vi "RunTest.vi"(8 "error in (no error)":errorcluster, 11 "Prueba09 in":refnum<class "Prueba09.lvclass">) -> (0 "error out":errorcluster, 2 "resultado":string, 3 "Prueba09 out":refnum<class "Prueba09.lvclass">)   [LabVIEW 2019, in "Prueba09.lvclass"]
uses:
  Prueba09.lvclass
  Prueba04/Control/Slide.ctl
  Prueba09.lvclass/Prueba09.ctl
  ClusterGEN.ctl
  <vilib>/Utility/miscctls.llb/LVRowAndColumnTypeDef.ctl
  <vilib>/Utility/error.llb/DialogType.ctl
  QMH/Message Queue/Enqueue Message (Single).vi
  <vilib>/Utility/error.llb/Error Cluster From Error Code.vi
  <vilib>/ErrorRing/Error Ring.xnode
  Prueba/Prueba.lvclass
  QMH/User Event - Stop/User Event - Stop.lvlib
  QMH/Message Queue/Message Queue.lvlib
  Prueba04/Prueba04.lvclass
panel:
  out "elapsed time":dbl
  out "cuenta":i32
  out "tablaPeakRef[dB]":string[](array[string])
  out "Vref2":dbl
  out "Pict Ring 2":u16(ring)
  out "Pict Ring 3":u16(ring)
  out "cumple_no_cumple":bool
  out "Vref":dbl
  in  "Tab":enum32{"Page 1", "Page 2", "Page 3"}(tab)
  out "NivMaxCpeak":dbl
  out "NivelRMSensayo":dbl
  out "frecuencia1":dbl
  in  "guardar_Vref":bool
  in  "generar1":bool
  in  "AjusteAmp":T1=40.0 caption="Ajuste de amplitud [mV]" scale=0.0..6000.0
  out "voltMon1":dbl format="%#.1f"
  out "frecMon1":dbl format="%#.1f"
  in  "seguir":bool
  out "NivMaxCpeak2":dbl
  out "NivelRMSensayo2":dbl
  out "frecuencia2":dbl
  in  "guardar_Vref2":bool
  in  "generar2":bool
  in  "AjusteAmp2":T1=40.0 caption="Ajuste de amplitud [mV]" scale=0.0..6000.0
  out "voltMon2":dbl format="%#.1f"
  out "frecMon2":dbl format="%#.1f"
  in  "seguir2":bool
  out "Pict Ring 4":u16(ring)
  out "Pict Ring 1":u16(ring)
  out "led":bool
  in  "knobFrec":dbl(knob)=1.0 min=1.0 max=3.0 scale=1.0..3.0
  in  "genera3":bool caption="PruebaSup"
  out "voltMon500":dbl format="%.1f"
  out "nivelRMS500":dbl format="%#.1f"
  in  "Tabla":string[][](table)
  in  "salir":bool
  out "cumple":bool
  out "no_cumple":bool
  out "voltMon8000":dbl format="%#.1f"
  out "nivelRM8000":dbl format="%#.1f"
  # "5550"
  # "3950"
  # "Selección de Señal de referencia 8000 Hz"
  # "Elección Señal de Referencia\nsegún marca y modelo de sonómetro"
  # "Nivel RMS para Ensayo"
  # "Nivel Máximo Cpeak"
  # "Frecuencia"
  # "Monitoreo"
  # "Frecuencia"
  # "Hz"
  # "Voltaje"
  # "mV"
  # "9. Nivel de sonido con ponderación Cpeak. IEC 61672-3: 2006 Cláusula 17"
  # "Selección de Señal de referencia 500 Hz"
  # "Elección Señal de Referencia\nsegún marca y modelo de sonómetro"
  # "Nivel RMS para Ensayo"
  # "Nivel Máximo Cpeak"
  # "Frecuencia"
  # "Monitoreo"
  # "Frecuencia"
  # "Hz"
  # "Voltaje"
  # "mV"
  # "9. Nivel de sonido con ponderación Cpeak. IEC 61672-3: 2006 Cláusula 17"
  # "Tabla Resultados"
  # "Genera peak"
  # "Cumple"
  # "No Cumple"
  # "500 Hz"
  # "Nivel RMS para Ensayo"
  # "dB"
  # "Voltaje"
  # "mV"
  # "9. Nivel de sonido con ponderación Cpeak. IEC 61672-3: 2006 Cláusula 17"
  # "8000 Hz"
  # "Nivel RMS para Ensayo"
  # "dB"
  # "Voltaje"
  # "mV"
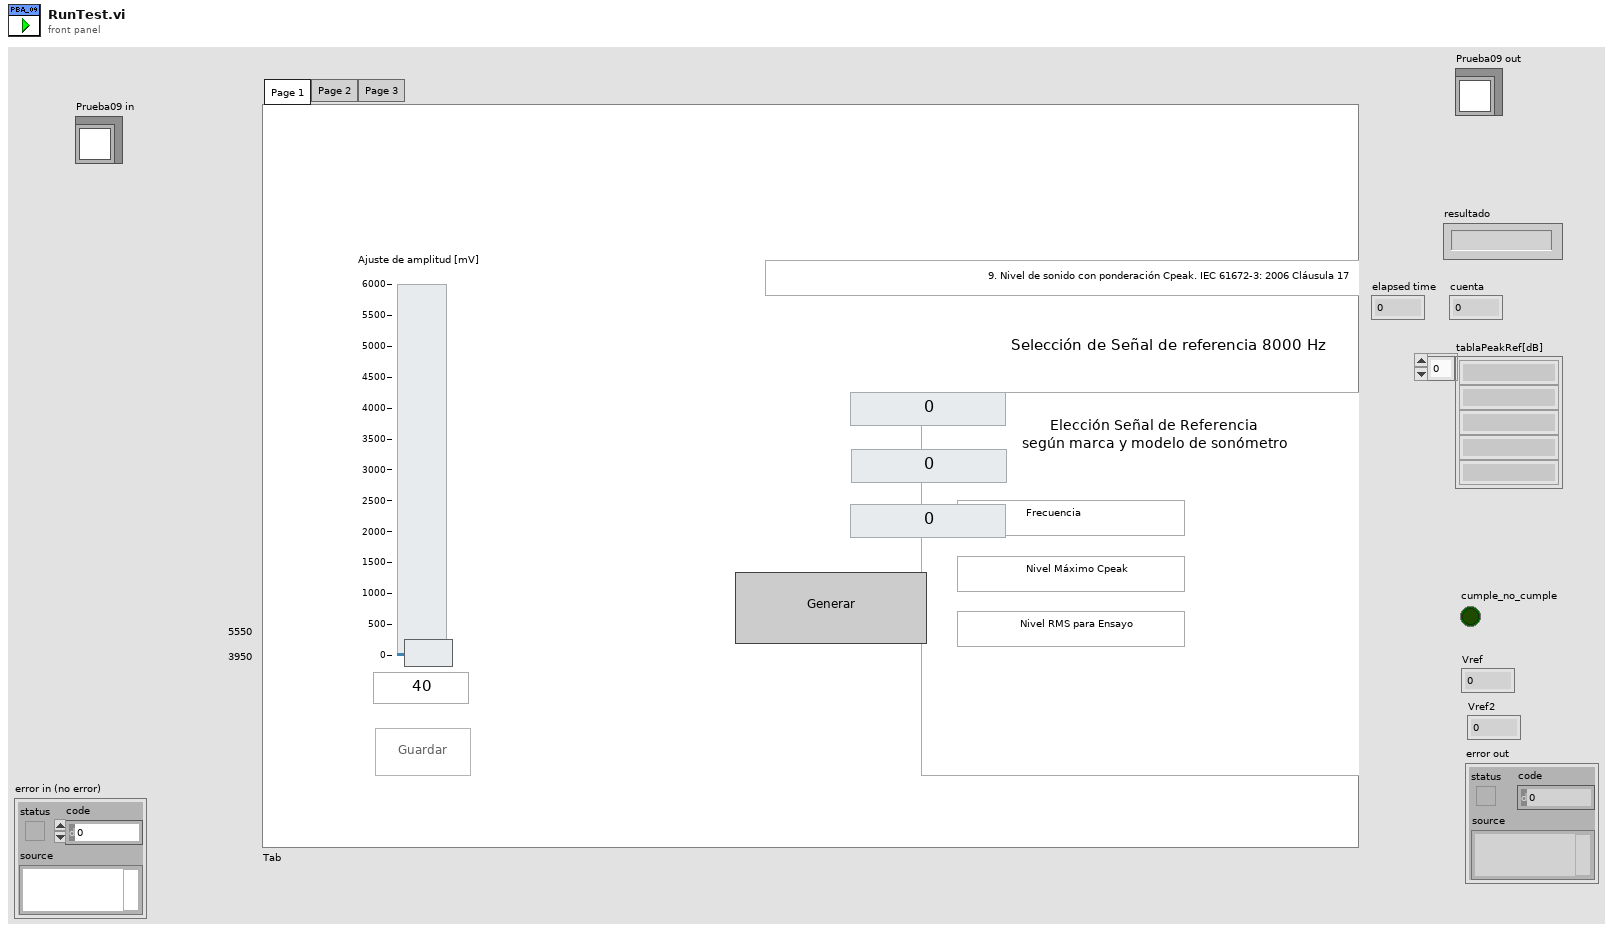
[diagram p1: front panel]
types:
  T1 = typedef "Prueba04.lvclass/Slide.ctl" = dbl
  T2 = typedef "LVRowAndColumnTypeDef.ctl" = cluster{"Row":i32, "Column":i32}
  T3 = typedef "Message Queue.lvlib/All Message Queues.ctl" = cluster{"MHL":refnum<queue>, "Inst_CNT90":refnum<queue>, "Inst_DS360":refnum<queue>, "Inst_Keithley2002":refnum<queue>, "Inst_DAQ":refnum<queue>, "BD":refnum<queue>, "Pistofono":refnum<queue>, "Nexus":refnum<queue>}
  T4 = enum8{"Enabled", "Disabled", "Disabled and Grayed Out"}
  T5 = enum32{"Page 1", "Page 2", "Page 3", "Page 4", "Page 5", "Page 6", "Page 7"}
  T6 = typedef "Prueba09.lvclass/ClusterGEN.ctl" = cluster{"frec":dbl, "amp":dbl, "tipo_ciclo":string}
  T7 = cluster{"ControlName":string, "ControlReference":refnum<vi>}[]
  T8 = typedef "DialogType.ctl" = u16
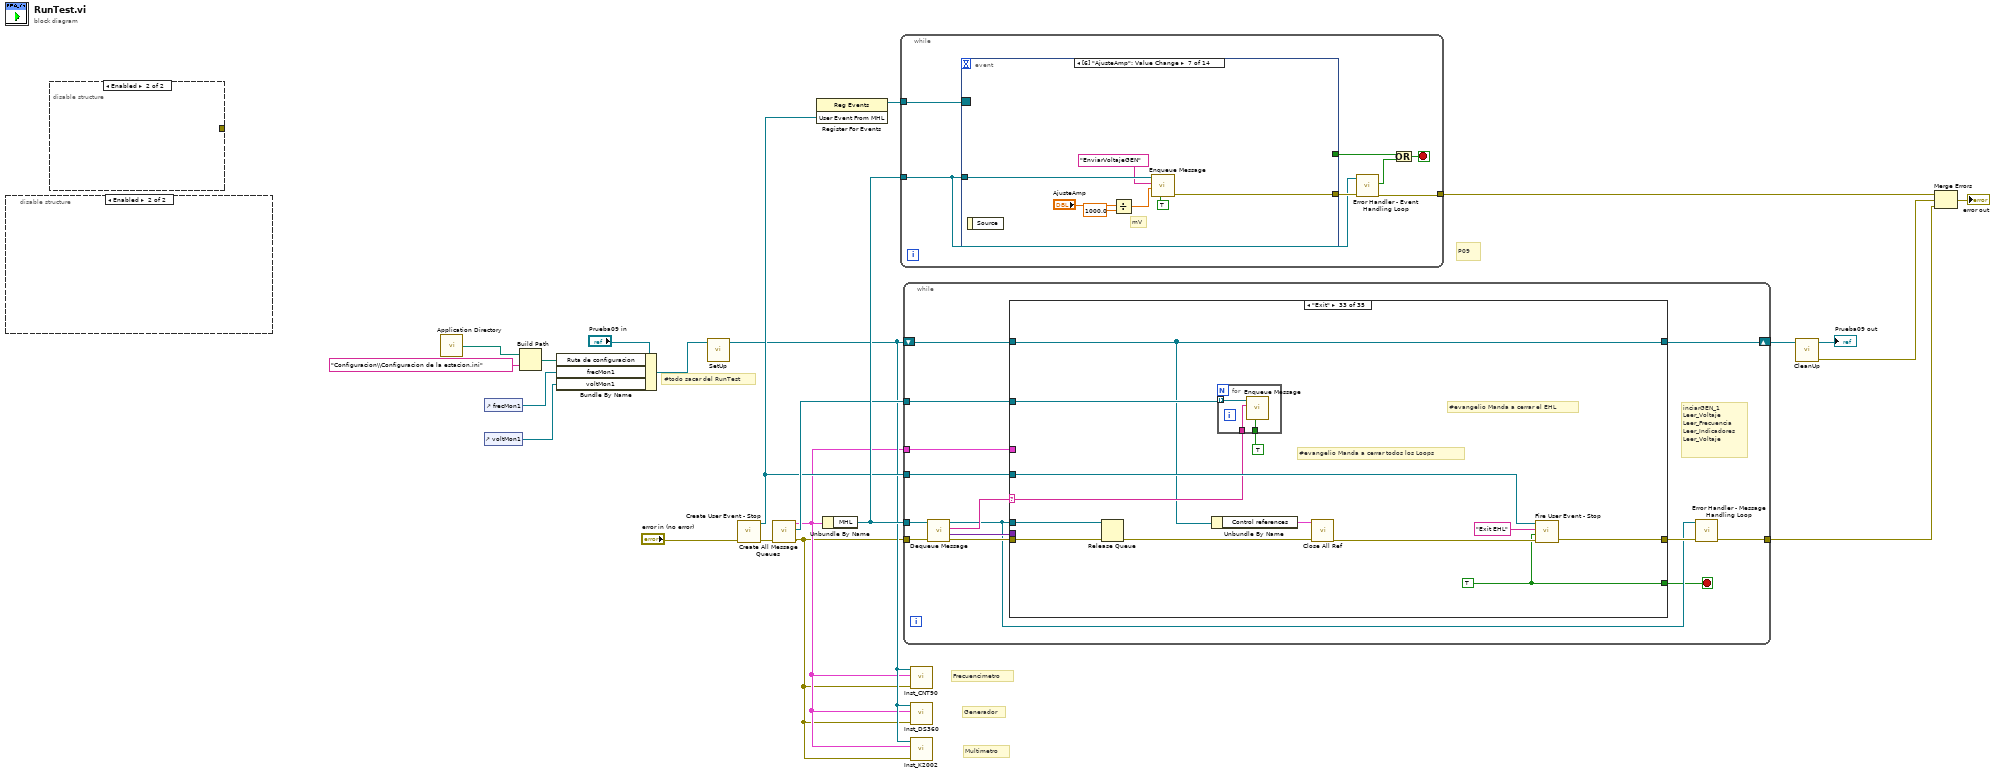
[diagram p0: block diagram]
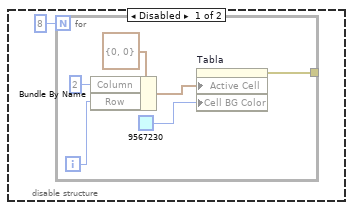
[diagram p2: hidden frame]
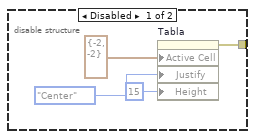
[diagram p3: hidden frame]
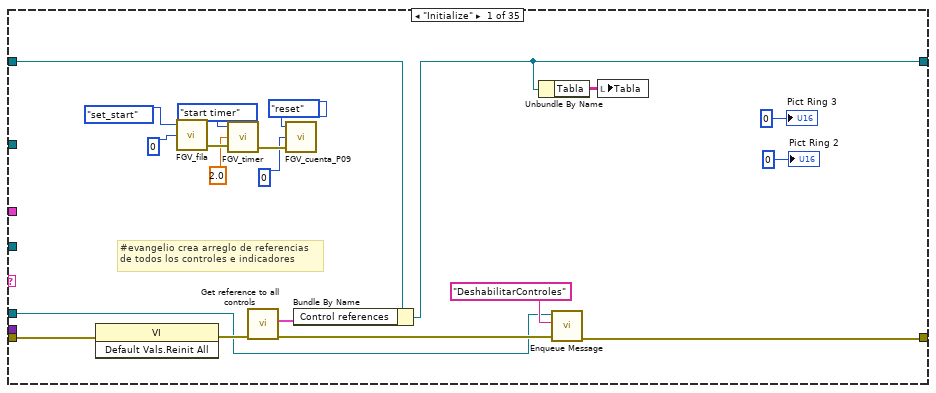
[diagram p4: hidden frame]
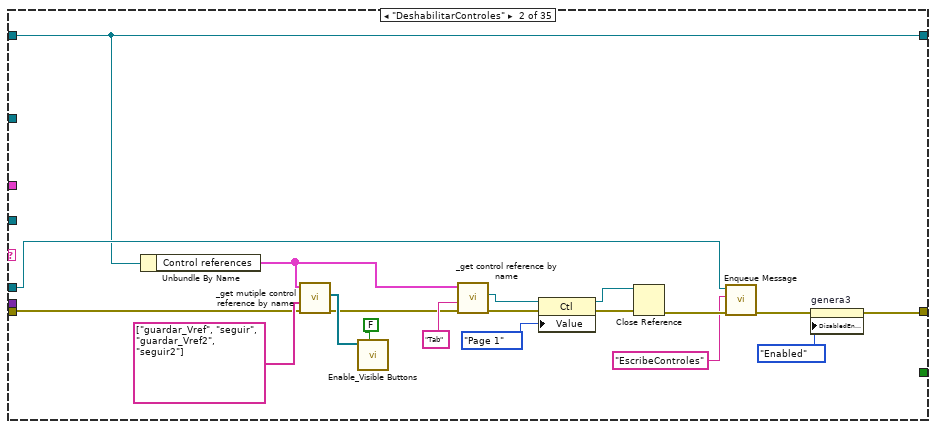
[diagram p5: hidden frame]
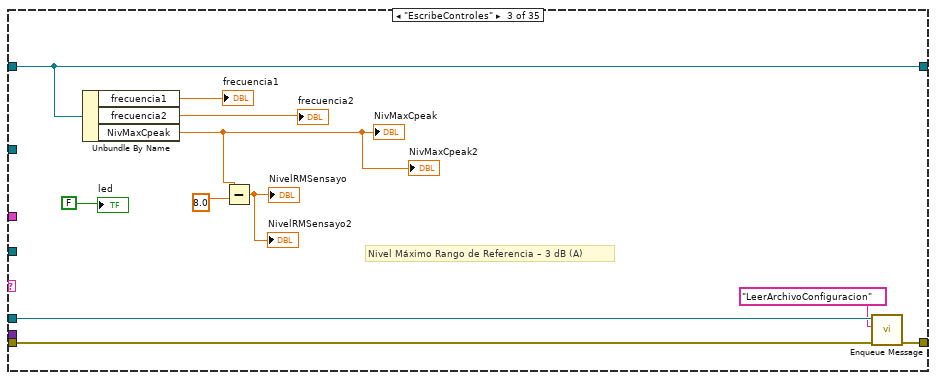
[diagram p6: hidden frame]
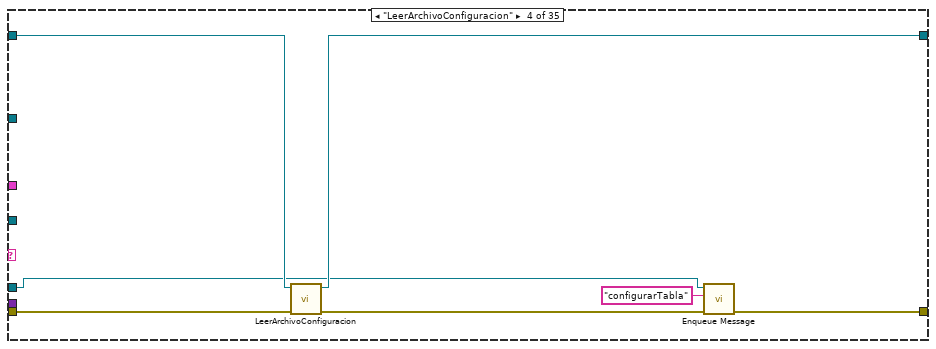
[diagram p7: hidden frame]
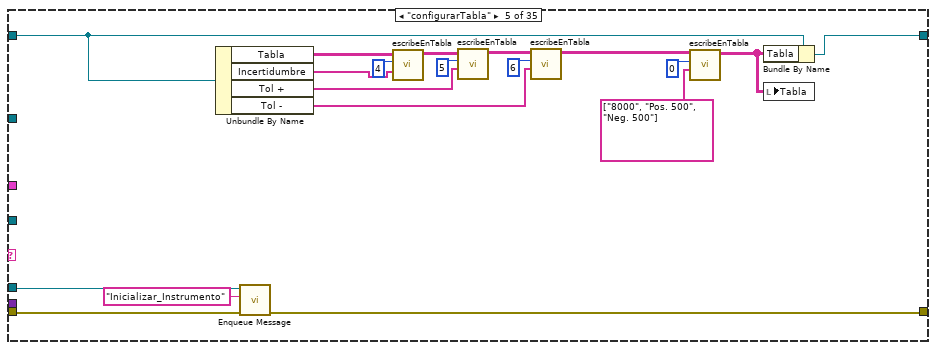
[diagram p8: hidden frame]
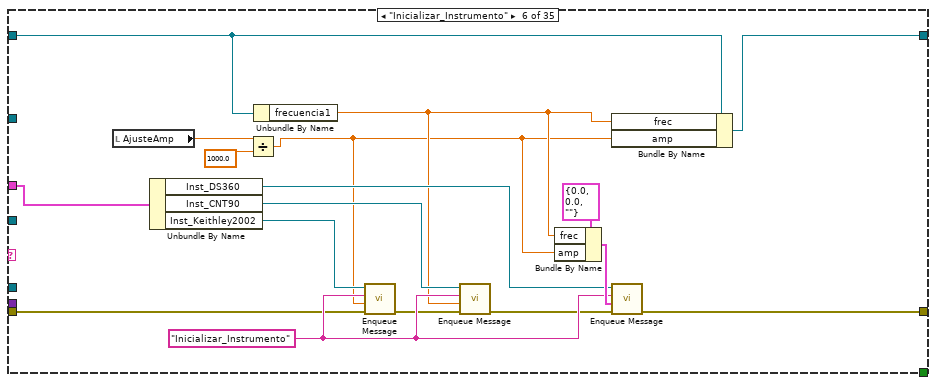
[diagram p9: hidden frame]
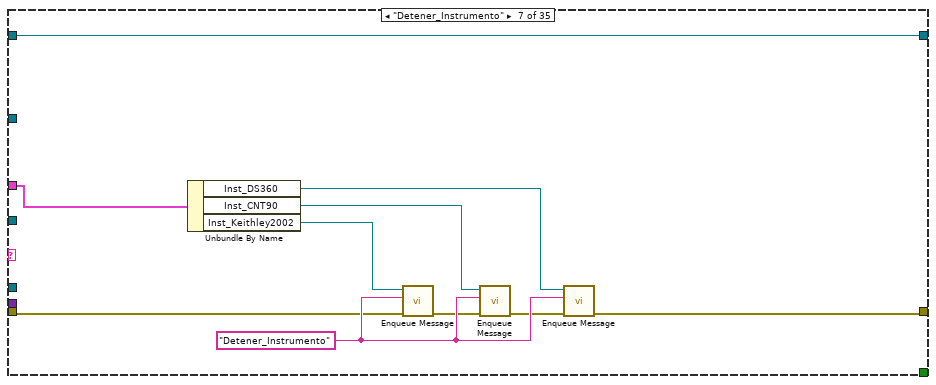
[diagram p10: hidden frame]
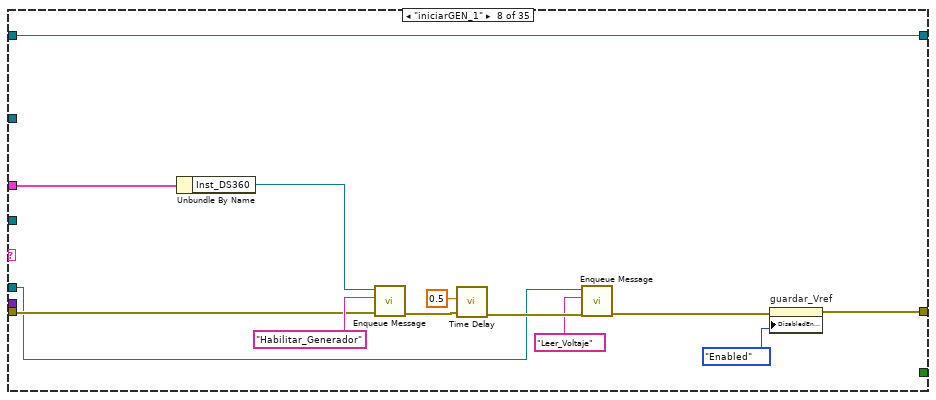
[diagram p11: hidden frame]
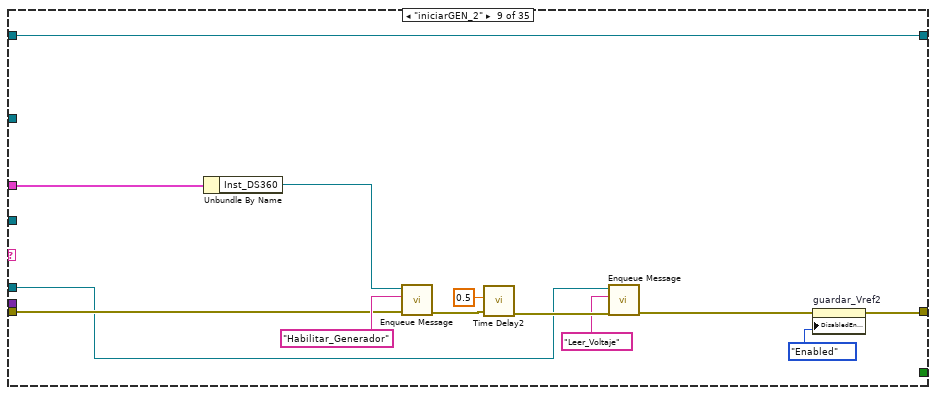
[diagram p12: hidden frame]
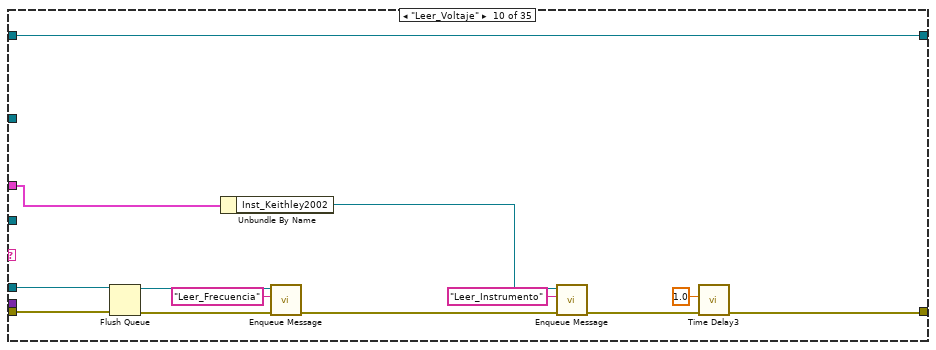
[diagram p13: hidden frame]
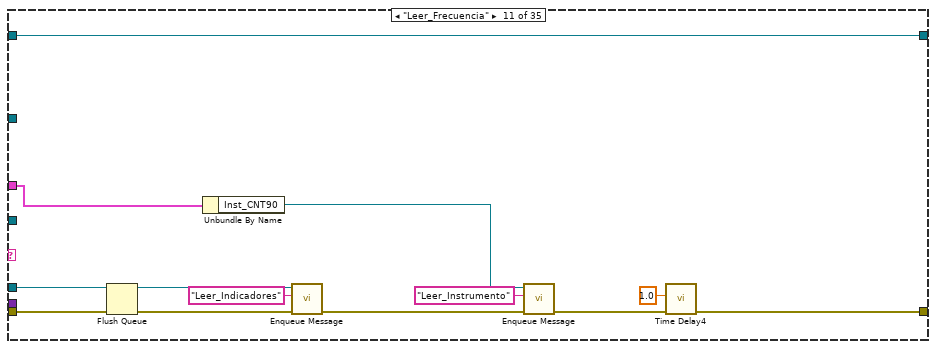
[diagram p14: hidden frame]
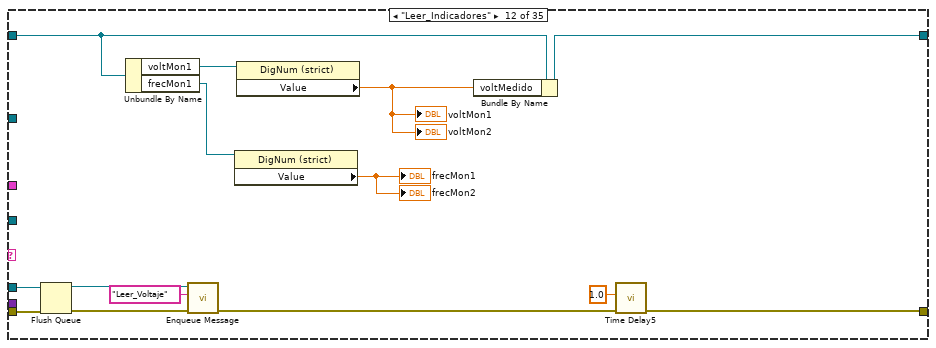
[diagram p15: hidden frame]
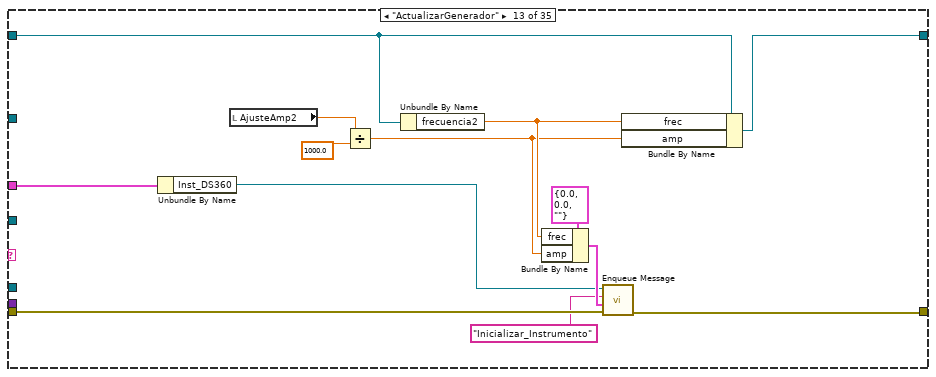
[diagram p16: hidden frame]
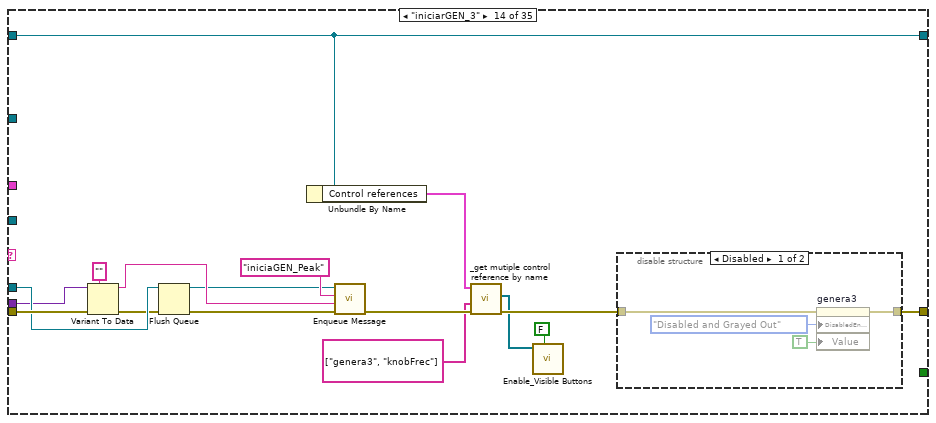
[diagram p17: hidden frame]
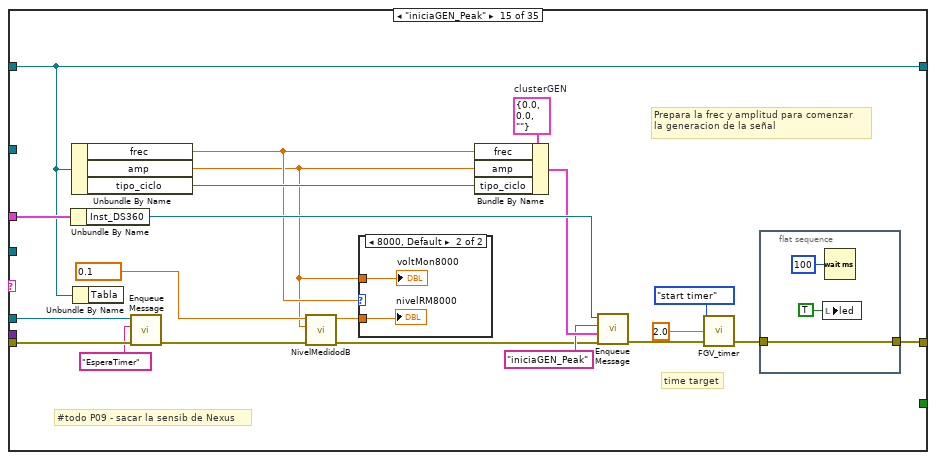
[diagram p19: hidden frame]
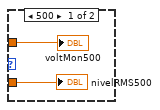
[diagram p20: hidden frame]
diagram:
  # "Multimetro"
  # "Generador"
  # "Frecuencimetro"
  # "P09"
  # "#todo sacar del RunTest"
  n1 = disable-structure shown="Enabled" {
    frame Disabled {
      n2 = for {
        N: 8 -> [_]
        tunnel: [w25] -> _
        i -> [w24]
        n3 = Bundle By Name(cluster=T2 {"Row"=0, "Column"=0} ("Active Cell:Active Cell"), "Column"=2, "Row"=w24) -> (w27:T2)
        n4 = property on="Tabla" class="Tbl (strict)"("Active Cell"=w27, "Cell BG Color"=u32 9567230) -> (error out=w25:errorcluster)  [unwired: 2 in, 1 out]
      }
    }
    frame Enabled {
    }
  }
  n5 = disable-structure shown="Enabled" {
    disable-tunnel: [w32 _] -> _
    frame Disabled {
      n6 = property on="Tabla" class="Tbl (strict)"("Active Cell"=T2 {"Row"=-2, "Column"=-2} ("Active Cell:Active Cell"), "Justify"=enum16{"Left", "Center", "Right"}."Center" ("Active Cell:Cell Justification"), "Height"=u32 15 ("Active Cell:Cell Font:Size")) -> (error out=w32:errorcluster)  [unwired: 2 in, 1 out]
    }
    frame Enabled {
    }
  }
  n7 = call <vilib>:"Application Directory.vi"() -> ("Application Directory"=w19:path)
  n8 = control-ref of="frecMon1"() -> (w6:refnum<vi>)
  n9 = control-ref of="voltMon1"() -> (w5:refnum<vi>)
  n10 = Build Path(base path=w19, name or relative path="Configuracion\\Configuracion de la estacion.ini") -> (appended path=w16:path)
  n11 = Bundle By Name(cluster="Prueba09 in", "Ruta de configuracion"=w16, "frecMon1"=w6, "voltMon1"=w5) -> (w17:refnum<class "Prueba09.lvclass">)
  n12 = call-dynamic "SetUp.vi"("Prueba08 in"=w17) -> ("Prueba08 out"=w9:refnum<class "Prueba09.lvclass">)  [unwired: 9 in, 1 out]
  n13 = call "Create User Event - Stop.vi"("error in (no error)"="error in (no error)") -> ("error out"=w15:errorcluster, "User Event From MHL"=w10:refnum<user-event>)  [unwired: 9 in]
  n14 = call "Create All Message Queues.vi"("error in (no error)"=w15) -> ("error out"=w7:errorcluster, "PL Queues Array"=w11:refnum<queue>[], "All Message Queues out"=w8:T3)  [unwired: 8 in]
  n15 = register-events(w10) -> (reference out=w12:refnum<event-registration>)  [unwired: 2 in, 1 out]
  n16 = Unbundle By Name(w8) -> ("MHL"=w13:refnum<queue>)
  n17 = while {
    tunnel: w13 -> [w35]
    tunnel: [w37] -> w22
    tunnel: w12 -> [w39]
    stop <- w40 stop-if-true
    n18 = event shown="[6] \"AjusteAmp\": Value Change" {
      selector: w39 -> [_ _ _ _ _ _ _ _ _ _ _ _ _ _]
      dyn-events: _ -> [_ _ _ _ _ _ _ _ _ _ _ _ _ _]
      timeout: _ -> [_ _ _ _ _ _ _ _ _ _ _ _ _ _]
      tunnel: w35 -> [w43 w49 w57 w62 w68 w75 w81 w84 w94 w101 w109 _ w117 w121]
      tunnel: [w42 w50 w56 w63 w70 w71 w82 w86 w91 w97 w104 _ _ w120] -> w38
      tunnel: [_ _ _ _ _ _ _ _ _ _ _ w110 _ _] -> w34
      event "salir": Value Change {
        n19 = event-data() -> ()  [unwired: 1 in, 1 out]
        n20 = call-poly "Enqueue Message.vi"("Message"="Exit", "Message Queue"=w43) -> ("error out"=w42:errorcluster)  [unwired: 8 in, 1 out]
      }
      event "generar1": Value Change {
        n21 = event-data() -> ("NewVal"=w46:bool)  [unwired: 1 in]
        n22 = Select(t="iniciarGEN_1", s=w46, f="detenerGEN") -> (s? t:f=w45:string)
        n23 = call-poly "Enqueue Message.vi"("Priority Message? (F)"=TRUE, "Message"=w45, "Message Queue"=w49) -> ("error out"=w50:errorcluster)  [unwired: 7 in, 1 out]
      }
      event "generar2": Value Change {
        n24 = event-data() -> ("NewVal"=w54:bool)  [unwired: 1 in]
        n25 = Select(t="iniciarGEN_2", s=w54, f="detenerGEN") -> (s? t:f=w52:string)
        n26 = call-poly "Enqueue Message.vi"("Priority Message? (F)"=TRUE, "Message"=w52, "Message Queue"=w57) -> ("error out"=w56:errorcluster)  [unwired: 7 in, 1 out]
      }
      event "genera3": Value Change {
        n27 = event-data() -> ()  [unwired: 1 in, 1 out]
        n28 = local read "knobFrec"() -> (w61:dbl)
        n29 = case shown="1" w61 {
          tunnel: ["Gen3_8000" "Gen3_500"] -> w60
          frame 1 {
          }
          frame Default {
          }
        }
        n30 = call-poly "Enqueue Message.vi"("Priority Message? (F)"=TRUE, "Message Data"=w60, "Message"="iniciarGEN_3", "Message Queue"=w62) -> ("error out"=w63:errorcluster)  [unwired: 6 in, 1 out]
      }
      event "seguir": Value Change {
        n31 = event-data() -> ()  [unwired: 1 in, 1 out]
        n32 = call-poly "Enqueue Message.vi"("Message"="ActualizarGenerador", "Message Queue"=w68) -> ("error out"=w67:errorcluster)  [unwired: 8 in, 1 out]
        n33 = property on="Tab" class="TabCtl (strict)"(error in=w67, "Value"=enum32{"Page 1", "Page 2", "Page 3"}."Page 2" ("Tab")) -> (error out=w70:errorcluster)  [unwired: 1 in, 1 out]
      }
      event "seguir2": Value Change {
        n34 = event-data() -> ()  [unwired: 1 in, 1 out]
        n35 = call-poly "Enqueue Message.vi"("Message"="peakRefer", "Message Queue"=w75) -> ("error out"=w72:errorcluster)  [unwired: 8 in, 1 out]
        n36 = property on="Tab" class="TabCtl (strict)"(error in=w72, "Value"=enum32{"Page 1", "Page 2", "Page 3"}."Page 3" ("Tab")) -> (error out=w71:errorcluster)  [unwired: 1 in, 1 out]
      }
      event Value Change {
        # "mV"
        n37 = event-data() -> ()  [unwired: 1 in, 1 out]
        n38 = Divide(x="AjusteAmp", y=T1 1000.0) -> (x/y=w77:T1)
        n39 = call-poly "Enqueue Message.vi"("Priority Message? (F)"=TRUE, "Message Data"=w77, "Message"="EnviarVoltajeGEN", "Message Queue"=w81) -> ("error out"=w82:errorcluster)  [unwired: 6 in, 1 out]
      }
      event Value Change {
        n40 = event-data() -> ()  [unwired: 1 in, 1 out]
        n41 = Divide(x="AjusteAmp2", y=T1 1000.0) -> (x/y=w87:T1)
        n42 = call-poly "Enqueue Message.vi"("Priority Message? (F)"=TRUE, "Message Data"=w87, "Message"="EnviarVoltajeGEN", "Message Queue"=w84) -> ("error out"=w86:errorcluster)  [unwired: 6 in, 1 out]
      }
      event "guardar_Vref": Value Change {
        n43 = event-data() -> ()  [unwired: 1 in, 1 out]
        n44 = call-poly "Enqueue Message.vi"("Priority Message? (F)"=TRUE, "Message"="guardaVref", "Message Queue"=w94) -> ("error out"=w92:errorcluster)  [unwired: 7 in, 1 out]
        n45 = property on="seguir" class="Bool"(error in=w92, "DisabledEnum"=T4."Enabled" ("Disabled")) -> (error out=w91:errorcluster)  [unwired: 1 in, 1 out]
      }
      event "guardar_Vref2": Value Change {
        n46 = event-data() -> ()  [unwired: 1 in, 1 out]
        n47 = call-poly "Enqueue Message.vi"("Priority Message? (F)"=TRUE, "Message"="guardaVref2", "Message Queue"=w101) -> ("error out"=w98:errorcluster)  [unwired: 7 in, 1 out]
        n48 = property on="seguir2" class="Bool"(error in=w98, "DisabledEnum"=T4."Enabled" ("Disabled")) -> (error out=w97:errorcluster)  [unwired: 1 in, 1 out]
      }
      event "Tabla": Value Change {
        n49 = event-data() -> ("CtlRef"=w107:refnum<vi>)  [unwired: 1 in]
        n50 = property class="Tbl (strict)"(reference=w107) -> ("Selection Start"=w103:T2)  [unwired: 1 in, 2 out]
        n51 = call-poly "Enqueue Message.vi"("Message"="LeerTabla", "Message Queue"=w109) -> ("error out"=w105:errorcluster, "dup Message Queue"=w106:refnum<queue>)  [unwired: 8 in]
        n52 = call-poly "Enqueue Message.vi"("error in (no error)"=w105, "Message Data"=w103, "Message"="ingresaMediciones", "Message Queue"=w106) -> ("error out"=w104:errorcluster)  [unwired: 6 in, 1 out]
      }
      event User Event {
        n53 = event-data() -> ("User Event"=w112:string, "Event Data"=w111:variant)  [unwired: 1 in]
        n54 = case shown="\"Exit EHL\"" w112 {
          tunnel: w111 -> [_ w114]
          tunnel: [_ w113] -> w110
          frame Default {
          }
          frame "Exit EHL" {
            # "#evangelio Termina\nla ejecucion del EHL"
            n55 = Variant To Data(type=TRUE, Variant=w114) -> (data=w113:bool)  [unwired: 1 in, 1 out]
          }
        }
      }
      event Panel Close? {
        w116 = TRUE
        n56 = event-data() -> ()  [unwired: 1 in, 1 out]
        n57 = call-poly "Enqueue Message.vi"("Priority Message? (F)"=w116, "Message"="Confirmar Salida", "Message Queue"=w117) -> ()  [unwired: 7 in, 2 out]
        n58 = event-data("Discard?"=w116) -> ()  [unwired: 1 in, 1 out]
      }
      event "knobFrec": Value Change {
        n59 = event-data() -> ()  [unwired: 1 in, 1 out]
        n60 = call-poly "Enqueue Message.vi"("Message"="ActualizarFrecAmpPeak", "Message Queue"=w121) -> ("error out"=w120:errorcluster)  [unwired: 8 in, 1 out]
      }
    }
    n61 = call "Error Handler - Event Handling Loop.vi"("error in (no error)"=w38, "Message Queue"=w35) -> ("dup error in"=w37:errorcluster, "Error?"=w36:bool)  [unwired: 7 in, 1 out]
    n62 = Or(x=w34, y=w36) -> (x .or. y?=w40:bool)
  }
  n63 = while {
    tunnel: w13 -> [w130]
    tunnel: w7 -> [w129]
    tunnel: [w124] -> w2
    shift-right: [w134] -> w4
    shift-left: w9 -> [w135]
    tunnel: w8 -> [w133]
    tunnel: w11 -> [w132]
    tunnel: w10 -> [w131]
    stop <- w122 stop-if-true
    # "inciarGEN_1\nLeer_Voltaje\nLeer_Frecuencia\nLeer_Indicadores\nLeer_Voltaje"
    n64 = call "Dequeue Message.vi"("error in (no error)"=w129, "Message Queue"=w130) -> ("error out"=w128:errorcluster, "Message Data"=w126:variant, "Message"=w127:string, "dup Message Queue"=w123:refnum<queue>)  [unwired: 6 in]
    n65 = case shown="\"Exit\"" w127 {
      selector: w127 -> [_ _ _ _ _ _ _ _ _ _ _ _ _ _ _ _ _ _ _ _ _ _ _ _ _ _ _ _ _ _ _ _ w592 _ w622]
      tunnel: w126 -> [_ _ _ _ _ _ _ _ _ _ _ _ _ w330 _ w370 _ _ _ w422 _ _ _ _ _ w519 w528 _ _ _ w577 _ _ _ _]
      tunnel: w128 -> [w150 w161 w185 w192 w196 w219 w231 w242 w256 w268 w281 w298 w312 w334 w360 w371 w392 w400 w413 w427 w435 w444 w460 w471 w475 w520 w529 w540 w562 w571 w580 w588 w596 w607 _]
      tunnel: [w149 w157 w184 w188 w194 w221 w229 w249 w263 w266 w279 w297 w314 w325 w355 w368 w391 w400 w413 w426 w433 w443 w458 w471 w486 w514 w524 w536 w562 w571 w578 w588 w590 w605 w621] -> w125
      tunnel: w123 -> [w151 w160 w183 w187 w195 _ _ w239 w254 w265 w278 w299 _ w332 w347 _ w383 _ _ w424 w432 w442 w459 _ w474 _ _ w539 _ _ w579 _ w595 w606 _]
      tunnel: w135 -> [w138 w159 w181 w190 w204 w227 w238 w251 w252 w277 w290 w296 w316 w324 w342 w380 w390 w395 w412 w420 w431 w437 w455 w466 w473 w518 w527 w537 w563 w572 w586 w587 w591 w612 w623]
      tunnel: [w136 w159 w181 w191 w203 w228 w238 w251 w252 w277 w290 w293 w317 w324 w342 w380 w385 w396 w411 w414 w428 w437 w455 w466 w473 w517 w526 w537 w563 w572 w586 w587 w591 w612 w623] -> w134
      tunnel: w133 -> [_ _ _ _ _ w218 w230 w241 w255 w267 w280 _ w311 _ w354 w369 _ _ _ _ _ _ _ _ _ _ _ w538 _ _ _ _ _ _ _]
      tunnel: w132 -> [_ _ _ _ _ _ _ _ _ _ _ _ _ _ _ _ _ _ _ _ _ _ _ _ _ _ _ _ _ _ _ _ w594 _ _]
      tunnel: w131 -> [_ _ _ _ _ _ _ _ _ _ _ _ _ _ _ _ _ _ _ _ _ _ _ _ _ _ _ _ _ _ _ _ w593 _ _]
      tunnel: [_ _ _ _ _ _ _ _ _ _ _ _ _ _ _ _ _ _ _ _ _ _ _ _ _ _ _ _ _ _ _ _ w589 _ _] -> w122
      frame "Initialize" {
        # "#evangelio crea arreglo de referencias\nde todos los controles e indicadores"
        n66 = invoke class="VI" method="Default Vals.Reinit All"(error in=w150) -> (error out=w154:errorcluster)  [unwired: 2 in, 2 out]
        n67 = call "FGV_fila.vi"("fila_inicial"=0, "action"=enum16{"increment", "set_start", "get"}."set_start") -> ("error out"=w148:errorcluster)  [unwired: 2 in, 1 out]
        n68 = call "FGV_timer.vi"("error in (no error)"=w148, "time target"=2.0, "action"=enum16{"get time", "start timer"}."start timer") -> ("error out"=w147:errorcluster)  [unwired: 2 out]
        n69 = call "Get reference to all controls.vi"("error in (no error)"=w154) -> ("error out"=w152:errorcluster, "Control references"=w153:T7)  [unwired: 5 in]
        n70 = call "FGV_cuenta_P09.vi"("error in (no error)"=w147, "cuenta in"=0, "action"=enum16{"increment", "reset", "get"}."reset") -> ()  [unwired: 1 in, 2 out]
        n71 = Bundle By Name(cluster=w138, "Control references"=w153) -> (w136:refnum<class "Prueba09.lvclass">)
        n72 = Unbundle By Name(w136) -> ("Tabla"=w137:string[][])
        n73 = call-poly "Enqueue Message.vi"("error in (no error)"=w152, "Message"="DeshabilitarControles", "Message Queue"=w151) -> ("error out"=w149:errorcluster)  [unwired: 7 in, 1 out]
        n74 = local write "Tabla"(w137) -> ()
        "Pict Ring 2" <- u16 0 ("Pict Ring 2")
        "Pict Ring 3" <- u16 0 ("Pict Ring 3")
      }
      frame "DeshabilitarControles" {
        n75 = Unbundle By Name(w159) -> ("Control references"=w170:T7)
        n76 = call "_get mutiple control reference by name.vi"("error in (no error)"=w161, "Control names"=string[] ["guardar_Vref", "seguir", "guardar_Vref2", "seguir2"], "Control references"=w170) -> ("error out"=w167:errorcluster, "References"=w168:refnum<vi>[])  [unwired: 3 in]
        n77 = call "Enable_Visible Buttons.vi"("Enable? (T)"=FALSE, "Controls Ref Array"=w168) -> ()  [unwired: 10 in]
        n78 = call "_get control reference by name.vi"("error in (no error)"=w167, "Control name"="Tab" ("Message"), "Control references"=w170) -> ("error out"=w174:errorcluster, "Ctl Refnum"=w172:refnum<vi>)  [unwired: 3 in]
        n79 = property class="Ctl"(reference=w172, error in=w174, "Value"=T5."Page 1" ("Tab_Prueba04")) -> (reference out=w163:refnum<vi>, error out=w165:errorcluster)
        n80 = Close Reference(reference=w163, error in (no error)=w165) -> (error out=w164:errorcluster)
        n81 = call-poly "Enqueue Message.vi"("error in (no error)"=w164, "Message"="EscribeControles", "Message Queue"=w160) -> ("error out"=w158:errorcluster)  [unwired: 7 in, 1 out]
        n82 = property on="genera3" class="Bool (strict)"(error in=w158, "DisabledEnum"=T4."Enabled" ("Disabled")) -> (error out=w157:errorcluster)  [unwired: 1 in, 1 out]
      }
      frame "EscribeControles" {
        # "Nivel Máximo Rango de Referencia – 3 dB (A)"
        n83 = Unbundle By Name(w181) -> ("frecuencia1"=→"frecuencia1":dbl, "frecuencia2"=→"frecuencia2":dbl, "NivMaxCpeak"=w178:dbl)
        "NivMaxCpeak" <- w178
        "NivMaxCpeak2" <- w178
        n84 = Subtract(x=w178, y=8.0) -> (x-y=→"NivelRMSensayo" →"NivelRMSensayo2":dbl)
        n85 = call-poly "Enqueue Message.vi"("error in (no error)"=w185, "Message"="LeerArchivoConfiguracion", "Message Queue"=w183) -> ("error out"=w184:errorcluster)  [unwired: 7 in, 1 out]
        "led" <- FALSE ("led")
      }
      frame "LeerArchivoConfiguracion" {
        n86 = call "LeerArchivoConfiguracion.vi"("error in"=w192, "Prueba31 in"=w190) -> ("error out"=w189:errorcluster, "Prueba31 out"=w191:refnum<class "Prueba09.lvclass">)  [unwired: 8 in]
        n87 = call-poly "Enqueue Message.vi"("error in (no error)"=w189, "Message"="configurarTabla", "Message Queue"=w187) -> ("error out"=w188:errorcluster)  [unwired: 7 in, 1 out]
      }
      frame "configurarTabla" {
        n88 = Unbundle By Name(w204) -> ("Tabla"=w202:string[][], "Incertidumbre"=w201:string[], "Tol +"=w200:string[], "Tol -"=w199:string[])
        n89 = call-poly "Enqueue Message.vi"("error in (no error)"=w196, "Message"="Inicializar_Instrumento", "Message Queue"=w195) -> ("error out"=w194:errorcluster)  [unwired: 7 in, 1 out]
        n90 = call "escribeEnTabla.vi"("parametros"=w201, "col"=4, "tabla in"=w202) -> ("tabla out"=w211:string[][])  [unwired: 8 in]
        n91 = call "escribeEnTabla.vi"("parametros"=w200, "col"=5, "tabla in"=w211) -> ("tabla out"=w210:string[][])  [unwired: 8 in]
        n92 = call "escribeEnTabla.vi"("parametros"=w199, "col"=6, "tabla in"=w210) -> ("tabla out"=w206:string[][])  [unwired: 8 in]
        n93 = call "escribeEnTabla.vi"("parametros"=string[] ["8000", "Pos. 500", "Neg. 500"], "col"=0, "tabla in"=w206) -> ("tabla out"=w193:string[][])  [unwired: 8 in]
        n94 = Bundle By Name(cluster=w204, "Tabla"=w193) -> (w203:refnum<class "Prueba09.lvclass">)
        n95 = local write "Tabla"(w193) -> ()
      }
      frame "Inicializar_Instrumento" {
        w224 = "Inicializar_Instrumento" ("Message")
        n96 = local read "AjusteAmp"() -> (w214:T1)
        n97 = Unbundle By Name(w218) -> ("Inst_DS360"=w216:refnum<queue>, "Inst_CNT90"=w220:refnum<queue>, "Inst_Keithley2002"=w226:refnum<queue>)
        n98 = Divide(x=w214, y=T1 1000.0) -> (x/y=w212:T1)
        n99 = Unbundle By Name(w227) -> ("frecuencia1"=w215:dbl)
        n100 = call-poly "Enqueue Message.vi"("error in (no error)"=w219, "Message Data"=w212, "Message"=w224, "Message Queue"=w226) -> ("error out"=w223:errorcluster)  [unwired: 6 in, 1 out]
        n101 = call-poly "Enqueue Message.vi"("error in (no error)"=w223, "Message Data"=w215, "Message"=w224, "Message Queue"=w220) -> ("error out"=w222:errorcluster)  [unwired: 6 in, 1 out]
        n102 = Bundle By Name(cluster=T6 {"frec"=0.0, "amp"=0.0, "tipo_ciclo"=""} ("clusterGEN"), "frec"=w215, "amp"=w212) -> (w225:T6)
        n103 = Bundle By Name(cluster=w227, "frec"=w215, "amp"=w212) -> (w228:refnum<class "Prueba09.lvclass">)
        n104 = call-poly "Enqueue Message.vi"("error in (no error)"=w222, "Message Data"=w225, "Message"=w224, "Message Queue"=w216) -> ("error out"=w221:errorcluster)  [unwired: 6 in, 1 out]
      }
      frame "Detener_Instrumento" {
        w234 = "Detener_Instrumento" ("Message")
        n105 = Unbundle By Name(w230) -> ("Inst_DS360"=w237:refnum<queue>, "Inst_CNT90"=w236:refnum<queue>, "Inst_Keithley2002"=w235:refnum<queue>)
        n106 = call-poly "Enqueue Message.vi"("error in (no error)"=w231, "Message"=w234, "Message Queue"=w235) -> ("error out"=w233:errorcluster)  [unwired: 7 in, 1 out]
        n107 = call-poly "Enqueue Message.vi"("error in (no error)"=w233, "Message"=w234, "Message Queue"=w236) -> ("error out"=w232:errorcluster)  [unwired: 7 in, 1 out]
        n108 = call-poly "Enqueue Message.vi"("error in (no error)"=w232, "Message"=w234, "Message Queue"=w237) -> ("error out"=w229:errorcluster)  [unwired: 7 in, 1 out]
      }
      frame "iniciarGEN_1" {
        n109 = Unbundle By Name(w241) -> ("Inst_DS360"=w247:refnum<queue>)
        n110 = call-poly "Enqueue Message.vi"("error in (no error)"=w242, "Message"="Habilitar_Generador", "Message Queue"=w247) -> ("error out"=w245:errorcluster)  [unwired: 7 in, 1 out]
        n111 = call "Time Delay"("error in (no error)"=w245, "Delay Time (s)"=0.5) -> ("error out"=w244:errorcluster)  [unwired: 9 in]
        n112 = call-poly "Enqueue Message.vi"("error in (no error)"=w244, "Message"="Leer_Voltaje", "Message Queue"=w239) -> ("error out"=w240:errorcluster)  [unwired: 7 in, 1 out]
        n113 = property on="guardar_Vref" class="Bool"(error in=w240, "DisabledEnum"=T4."Enabled" ("Disabled")) -> (error out=w249:errorcluster)  [unwired: 1 in, 1 out]
      }
      frame "iniciarGEN_2" {
        n114 = Unbundle By Name(w255) -> ("Inst_DS360"=w261:refnum<queue>)
        n115 = call-poly "Enqueue Message.vi"("error in (no error)"=w256, "Message"="Habilitar_Generador", "Message Queue"=w261) -> ("error out"=w259:errorcluster)  [unwired: 7 in, 1 out]
        n116 = call "Time Delay2"("error in (no error)"=w259, "Delay Time (s)"=0.5) -> ("error out"=w258:errorcluster)  [unwired: 9 in]
        n117 = call-poly "Enqueue Message.vi"("error in (no error)"=w258, "Message"="Leer_Voltaje", "Message Queue"=w254) -> ("error out"=w253:errorcluster)  [unwired: 7 in, 1 out]
        n118 = property on="guardar_Vref2" class="Bool"(error in=w253, "DisabledEnum"=T4."Enabled" ("Disabled")) -> (error out=w263:errorcluster)  [unwired: 1 in, 1 out]
      }
      frame "Leer_Voltaje" {
        n119 = Flush Queue(queue=w265, error in (no error)=w268) -> (queue out=w269:refnum<queue>, error out=w270:errorcluster)  [unwired: 1 out]
        n120 = Unbundle By Name(w267) -> ("Inst_Keithley2002"=w273:refnum<queue>)
        n121 = call-poly "Enqueue Message.vi"("error in (no error)"=w270, "Message"="Leer_Frecuencia", "Message Queue"=w269) -> ("error out"=w276:errorcluster)  [unwired: 7 in, 1 out]
        n122 = call-poly "Enqueue Message.vi"("error in (no error)"=w276, "Message"="Leer_Instrumento", "Message Queue"=w273) -> ("error out"=w274:errorcluster)  [unwired: 7 in, 1 out]
        n123 = call "Time Delay3"("error in (no error)"=w274, "Delay Time (s)"=1.0) -> ("error out"=w266:errorcluster)  [unwired: 9 in]
      }
      frame "Leer_Frecuencia" {
        n124 = Flush Queue(queue=w278, error in (no error)=w281) -> (queue out=w282:refnum<queue>, error out=w283:errorcluster)  [unwired: 1 out]
        n125 = Unbundle By Name(w280) -> ("Inst_CNT90"=w286:refnum<queue>)
        n126 = call-poly "Enqueue Message.vi"("error in (no error)"=w283, "Message"="Leer_Indicadores", "Message Queue"=w282) -> ("error out"=w289:errorcluster)  [unwired: 7 in, 1 out]
        n127 = call-poly "Enqueue Message.vi"("error in (no error)"=w289, "Message"="Leer_Instrumento", "Message Queue"=w286) -> ("error out"=w287:errorcluster)  [unwired: 7 in, 1 out]
        n128 = call "Time Delay4"("error in (no error)"=w287, "Delay Time (s)"=1.0) -> ("error out"=w279:errorcluster)  [unwired: 9 in]
      }
      frame "Leer_Indicadores" {
        n129 = Flush Queue(queue=w299, error in (no error)=w298) -> (queue out=w300:refnum<queue>, error out=w301:errorcluster)  [unwired: 1 out]
        n130 = Unbundle By Name(w296) -> ("voltMon1"=w295:refnum<vi>, "frecMon1"=w294:refnum<vi>)
        n131 = call-poly "Enqueue Message.vi"("error in (no error)"=w301, "Message"="Leer_Voltaje", "Message Queue"=w300) -> ("error out"=w304:errorcluster)  [unwired: 7 in, 1 out]
        n132 = property class="DigNum (strict)"(reference=w294) -> ("Value"=→"frecMon2" →"frecMon1":dbl)  [unwired: 1 in, 2 out]
        n133 = property class="DigNum (strict)"(reference=w295) -> ("Value"=w291:dbl)  [unwired: 1 in, 2 out]
        "voltMon2" <- w291
        "voltMon1" <- w291
        n134 = Bundle By Name(cluster=w296, "voltMedido"=w291) -> (w293:refnum<class "Prueba09.lvclass">)
        n135 = call "Time Delay5"("error in (no error)"=w304, "Delay Time (s)"=1.0) -> ("error out"=w297:errorcluster)  [unwired: 9 in]
      }
      frame "ActualizarGenerador" {
        n136 = Unbundle By Name(w311) -> ("Inst_DS360"=w313:refnum<queue>)
        n137 = local read "AjusteAmp2"() -> (w308:T1)
        n138 = Divide(x=w308, y=T1 1000.0) -> (x/y=w306:T1)
        n139 = Unbundle By Name(w316) -> ("frecuencia2"=w309:dbl)
        n140 = Bundle By Name(cluster=T6 {"frec"=0.0, "amp"=0.0, "tipo_ciclo"=""} ("clusterGEN"), "frec"=w309, "amp"=w306) -> (w315:T6)
        n141 = call-poly "Enqueue Message.vi"("error in (no error)"=w312, "Message Data"=w315, "Message"="Inicializar_Instrumento", "Message Queue"=w313) -> ("error out"=w314:errorcluster)  [unwired: 6 in, 1 out]
        n142 = Bundle By Name(cluster=w316, "frec"=w309, "amp"=w306) -> (w317:refnum<class "Prueba09.lvclass">)
      }
      frame "iniciarGEN_3" {
        n143 = Variant To Data(error in=w334, type="", Variant=w330) -> (data=w327:string, error out=w331:errorcluster)
        n144 = Flush Queue(queue=w332, error in (no error)=w331) -> (queue out=w326:refnum<queue>, error out=w333:errorcluster)  [unwired: 1 out]
        n145 = Unbundle By Name(w324) -> ("Control references"=w323:T7)
        n146 = call-poly "Enqueue Message.vi"("error in (no error)"=w333, "Message Data"=w327, "Message"="iniciaGEN_Peak" ("tipo_ciclo"), "Message Queue"=w326) -> ("error out"=w322:errorcluster)  [unwired: 6 in, 1 out]
        n147 = call "_get mutiple control reference by name.vi"("error in (no error)"=w322, "Control names"=string[] ["genera3", "knobFrec"] ("tipo_ciclo"), "Control references"=w323) -> ("error out"=w321:errorcluster, "References"=w318:refnum<vi>[])  [unwired: 3 in]
        n148 = call "Enable_Visible Buttons.vi"("Enable? (T)"=FALSE, "Controls Ref Array"=w318) -> ()  [unwired: 10 in]
        n149 = disable-structure shown="Disabled" {
          disable-tunnel: [w338 w339] -> w325
          disable-tunnel: w321 -> [w335 w339]
          frame Disabled {
            n150 = property on="genera3" class="Bool (strict)"(error in=w335, "DisabledEnum"=T4."Disabled and Grayed Out" ("Disabled"), "Value"=TRUE ("genera3")) -> (error out=w338:errorcluster)  [unwired: 1 in, 1 out]
          }
          frame Enabled {
          }
        }
      }
      frame "iniciaGEN_Peak" {
        w341 = 0.1 items=["10m"=0.01, "31,6m"=0.0316, "100m"=0.1, "316m"=0.316, "1"=1.0] ("Sensibilidad")
        w352 = T6 {"frec"=0.0, "amp"=0.0, "tipo_ciclo"=""}  # clusterGEN
        # "#todo P09 - sacar la sensib de Nexus"
        # "time target"
        # "Prepara la frec y amplitud para comenzar\nla generacion de la señal"
        n151 = Unbundle By Name(w354) -> ("Inst_DS360"=w353:refnum<queue>)
        n152 = Unbundle By Name(w342) -> ("frec"=w343:dbl, "amp"=w340:dbl, "tipo_ciclo"=w351:string)
        n153 = Unbundle By Name(w342) -> ()  [unwired: 1 out]
        n154 = call-poly "Enqueue Message.vi"("error in (no error)"=w360, "Message"="EsperaTimer", "Message Queue"=w347) -> ("error out"=w348:errorcluster)  [unwired: 7 in, 1 out]
        n155 = call "NivelMedidodB.vi"("error in (no error)"=w348, "voltaje_medido"=w340, "Sensibilidad"=w341) -> ("error out"=w345:errorcluster, "Nivel Medido [dB]"=w344:dbl)  [unwired: 7 in]
        n156 = case shown="8000, Default" w343 {
          tunnel: w344 -> [w362 w364]
          tunnel: w340 -> [w361 w363]
          frame 500 {
            "nivelRMS500" <- w362
            "voltMon500" <- w361
          }
          frame 8000, Default {
            "voltMon8000" <- w363
            "nivelRM8000" <- w364
          }
        }
        n157 = Bundle By Name(cluster=w352, "frec"=w343, "amp"=w340, "tipo_ciclo"=w351) -> (w350:T6)
        n158 = call-poly "Enqueue Message.vi"("error in (no error)"=w345, "Message Data"=w350, "Message"="iniciaGEN_Peak", "Message Queue"=w353) -> ("error out"=w359:errorcluster)  [unwired: 6 in, 1 out]
        n159 = call "FGV_timer.vi"("error in (no error)"=w359, "time target"=2.0, "action"=enum16{"get time", "start timer"}."start timer") -> ("error out"=w356:errorcluster)  [unwired: 2 out]
        n160 = flat-sequence {
          tunnel: w356 -> [w367]
          tunnel: [w367] -> w355
          frame #0 {
            n161 = local write "led"(TRUE ("led")) -> ()
            n162 = Wait (ms)(milliseconds to wait=u32 100) -> ()  [unwired: 1 out]
          }
        }
      }
      frame "EnviarVoltajeGEN" {
        n163 = Unbundle By Name(w369) -> ("Inst_DS360"=w374:refnum<queue>, "Inst_Keithley2002"=w379:refnum<queue>)
        n164 = Variant To Data(error in=w371, type=0.0, Variant=w370) -> (data=w372:dbl, error out=w377:errorcluster)
        n165 = call-poly "Enqueue Message.vi"("error in (no error)"=w377, "Message Data"=w372, "Message"="ActualizarVoltaje", "Message Queue"=w379) -> ("error out"=w375:errorcluster)  [unwired: 6 in, 1 out]
        n166 = call-poly "Enqueue Message.vi"("error in (no error)"=w375, "Message Data"=w372, "Message"="ActualizarAmplitud", "Message Queue"=w374) -> ("error out"=w368:errorcluster)  [unwired: 6 in, 1 out]
      }
      frame "peakRefer" {
        # "Actualiza la frec y amplitud a enviar \nen el siguiente peak"
        n167 = call-poly "Enqueue Message.vi"("error in (no error)"=w392, "Message"="ActualizarFrecAmpPeak", "Message Queue"=w383) -> ("error out"=w384:errorcluster)  [unwired: 7 in, 1 out]
        n168 = call "peakRef.vi"("error in (no error)"=w384, "Prueba09 in"=w390) -> ("error out"=w391:errorcluster, "tablaPeakRef[dB]"=w386:string[], "Prueba09 out"=w389:refnum<class "Prueba09.lvclass">)  [unwired: 7 in]
        "tablaPeakRef[dB]" <- w386
        n169 = Unbundle By Name(w389) -> ("Tabla"=w388:string[][])
        n170 = call "escribeEnTabla.vi"("parametros"=w386, "col"=1, "tabla in"=w388) -> ("tabla out"=w381:string[][])  [unwired: 8 in]
        n171 = Bundle By Name(cluster=w389, "Tabla"=w381) -> (w385:refnum<class "Prueba09.lvclass">)
        n172 = local write "Tabla"(w381) -> ()
      }
      frame "ActualizarFrecAmpPeak" {
        # "solo pone los valores\npor defecto de estos controles\nen el cluster"
        n173 = To Long Integer(number="knobFrec") -> (32bit integer=w394:i32)
        n174 = case shown="3" w394 {
          tunnel: [8000.0 500.0 500.0] -> w399
          tunnel: [w402 w405 w408] -> w398
          tunnel: ["1" ("tipo_ciclo") ".5" ("tipo_ciclo") ".5" ("tipo_ciclo")] -> w397
          frame 1, Default {
            n175 = local read "Vref"() -> (w402:dbl)
          }
          frame 2 {
            n176 = local read "Vref2"() -> (w405:dbl)
          }
          frame 3 {
            n177 = local read "Vref2"() -> (w408:dbl)
          }
        }
        n178 = Bundle By Name(cluster=w395, "frec"=w399, "amp"=w398, "tipo_ciclo"=w397) -> (w396:refnum<class "Prueba09.lvclass">)
      }
      frame "LeerTabla" {
        n179 = Bundle By Name(cluster=w412, "Tabla"="Tabla") -> (w411:refnum<class "Prueba09.lvclass">)
      }
      frame "ingresaMediciones" {
        n180 = Flush Queue(queue=w424, error in (no error)=w427) -> (queue out=w423:refnum<queue>, error out=w425:errorcluster)  [unwired: 1 out]
        n181 = Variant To Data(error in=w425, type=T2 {"Row"=0, "Column"=0} ("Selection Start"), Variant=w422) -> (data=w416:T2, error out=w421:errorcluster)
        n182 = call "ingresaMediciones.vi"("error in (no error)"=w421, "Selection Start"=w416, "Prueba09 in"=w420) -> ("error out"=w419:errorcluster, "Prueba09 out"=w414:refnum<class "Prueba09.lvclass">)  [unwired: 7 in]
        n183 = Unbundle By Name(w414) -> ("Tabla"=w415:string[][])
        n184 = local write "Tabla"(w415) -> ()
        n185 = call-poly "Enqueue Message.vi"("error in (no error)"=w419, "Message"="cumplimiento", "Message Queue"=w423) -> ("error out"=w426:errorcluster)  [unwired: 7 in, 1 out]
      }
      frame "cumplimiento" {
        n186 = call "cumplimiento.vi"("error in (no error)"=w435, "Prueba09 in"=w431) -> ("error out"=w434:errorcluster, "Prueba09 out"=w428:refnum<class "Prueba09.lvclass">)  [unwired: 8 in]
        n187 = Unbundle By Name(w428) -> ("Tabla"=w429:string[][])
        n188 = local write "Tabla"(w429) -> ()
        n189 = call-poly "Enqueue Message.vi"("error in (no error)"=w434, "Message"="listo_evaluar", "Message Queue"=w432) -> ("error out"=w433:errorcluster)  [unwired: 7 in, 1 out]
      }
      frame "listo_evaluar" {
        n190 = Unbundle By Name(w437) -> ("Tabla"=w436:string[][])
        n191 = Index Array(array=w436, index (col)=7 ("disabled index (col)")) -> (element=w439:string[])  [unwired: 1 in]
        n192 = for {
          tunnel: [w452] -> w440 mode=indexing
          tunnel: w439 -> [w450] mode=indexing
          n193 = Not Equal?(x=w450, y="--") -> (x != y?=w452:bool)
        }
        n194 = And Array Elements(Boolean array=w440) -> (logical AND=w438:bool)
        n195 = case shown="True" w438 {
          tunnel: w444 -> [w445 w449]
          tunnel: [w445 w448] -> w443
          tunnel: w442 -> [_ w447]
          frame False {
          }
          frame True {
            n196 = call-poly "Enqueue Message.vi"("error in (no error)"=w449, "Message"="evaluar", "Message Queue"=w447) -> ("error out"=w448:errorcluster)  [unwired: 7 in, 1 out]
          }
        }
      }
      frame "evaluar" {
        # "si todos cumplen\nentonces el ensayo\ncumple"
        n197 = Unbundle By Name(w455) -> ("Tabla"=w454:string[][])
        n198 = call-poly "Enqueue Message.vi"("error in (no error)"=w460, "Message"="final", "Message Queue"=w459) -> ("error out"=w458:errorcluster)  [unwired: 7 in, 1 out]
        n199 = Index Array(array=w454, index (col)=7 ("disabled index (col)")) -> (element=w456:string[])  [unwired: 1 in]
        n200 = for {
          tunnel: [w465] -> w462 mode=indexing
          tunnel: w456 -> [w463] mode=indexing
          n201 = Equal?(x=w463, y="Cumple") -> (x = y?=w465:bool)
        }
        n202 = And Array Elements(Boolean array=w462) -> (logical AND=→"cumple_no_cumple":bool)
      }
      frame "final" {
        n203 = local read "cumple_no_cumple"() -> (w467:bool)
        "cumple" <- w467
        n204 = Not(x=w467) -> (.not. x?=→"no_cumple":bool)
        n205 = Select(t="Cumple", s=w467, f="No Cumple") -> (s? t:f=→"resultado":string)
      }
      frame "EsperaTimer" {
        n206 = call "FGV_timer.vi"("error in (no error)"=w475, "time target"=2.0, "action"=enum16{"get time", "start timer"}."get time") -> ("error out"=w483:errorcluster, "time elapsed?"=w484:bool, "elapsed time"=→"elapsed time":dbl)
        n207 = call "FGV_cuenta_P09.vi"("error in (no error)"=w483, "action"=enum16{"increment", "reset", "get"}."get") -> ("error out"=w476:errorcluster, "cuenta out"=w482:i32)  [unwired: 2 in]
        "cuenta" <- w482
        n208 = Greater Or Equal?(x=w482, y=9) -> (x >= y?=w480:bool)
        n209 = case shown="True" w484 {
          tunnel: [w492 w493] -> w486
          tunnel: w476 -> [w491 w499]
          tunnel: w480 -> [_ w498]
          tunnel: w474 -> [w490 w495]
          frame False {
            # "Aun no llegamos a los 2 segundos"
            n210 = call-poly "Enqueue Message.vi"("error in (no error)"=w491, "Message"="EsperaTimer", "Message Queue"=w490) -> ("error out"=w492:errorcluster)  [unwired: 7 in, 1 out]
            n211 = local write "led"(FALSE ("led")) -> ()
            n212 = Wait (ms)(milliseconds to wait=u32 250) -> ()  [unwired: 1 out]
          }
          frame True {
            # "Pasamos los 2 segundos"
            n213 = case shown="True" w498 {
              tunnel: [w501 w508] -> w494
              tunnel: w499 -> [w507 w513]
              tunnel: w495 -> [w504 w511]
              frame True {
                # "Pasamos los 10 pulsos"
                n214 = local write "genera3"(FALSE ("genera3")) -> ()
                n215 = call-poly "Enqueue Message.vi"("error in (no error)"=w507, "Message"="detenerGEN", "Message Queue"=w504) -> ("error out"=w502:errorcluster)  [unwired: 7 in, 1 out]
                n216 = call "FGV_cuenta_P09.vi"("error in (no error)"=w502, "cuenta in"=0, "action"=enum16{"increment", "reset", "get"}."reset") -> ("error out"=w501:errorcluster)  [unwired: 1 in, 1 out]
              }
              frame False {
                # "aun no llegamos a los 10 pulsos"
                n217 = call-poly "Enqueue Message.vi"("error in (no error)"=w513, "Message"="iniciaGEN_Peak", "Message Queue"=w511) -> ("error out"=w509:errorcluster)  [unwired: 7 in, 1 out]
                n218 = call "FGV_cuenta_P09.vi"("error in (no error)"=w509, "action"=enum16{"increment", "reset", "get"}."increment") -> ("error out"=w508:errorcluster)  [unwired: 2 in, 1 out]
              }
            }
            n219 = call "FGV_timer.vi"("error in (no error)"=w494, "time target"=2.0, "action"=enum16{"get time", "start timer"}."start timer") -> ("error out"=w493:errorcluster)  [unwired: 2 out]
          }
        }
      }
      frame "DatoRecibidoCNT90" {
        n220 = Variant To Data(error in=w520, type=0.0, Variant=w519) -> (data=w515:dbl, error out=w514:errorcluster)
        n221 = Bundle By Name(cluster=w518, "frecMedida"=w515) -> (w517:refnum<class "Prueba09.lvclass">)
      }
      frame "DatoRecibidoK2002" {
        n222 = Variant To Data(error in=w529, type=0.0, Variant=w528) -> (data=w522:dbl, error out=w524:errorcluster)
        n223 = Multiply(x=w522, y=1000.0) -> (x*y=w521:dbl)
        n224 = Bundle By Name(cluster=w527, "voltMedido"=w521) -> (w526:refnum<class "Prueba09.lvclass">)
      }
      frame "detenerGEN" {
        w553 = 0.0 ("voltaje1")
        n225 = Flush Queue(queue=w539, error in (no error)=w540) -> (error out=w542:errorcluster)  [unwired: 2 out]
        n226 = Unbundle By Name(w538) -> ("Inst_DS360"=w547:refnum<queue>)
        n227 = call "Time Delay7"("error in (no error)"=w542, "Delay Time (s)"=0.5) -> ("error out"=w541:errorcluster)  [unwired: 9 in]
        n228 = call-poly "Enqueue Message.vi"("error in (no error)"=w541, "Message"="Deshabilitar_Generador", "Message Queue"=w547) -> ("error out"=w546:errorcluster)  [unwired: 7 in, 1 out]
        n229 = call "Time Delay6"("error in (no error)"=w546, "Delay Time (s)"=0.5) -> ("error out"=w545:errorcluster)  [unwired: 9 in]
        n230 = Unbundle By Name(w537) -> ("Control references"=w530:T7)
        n231 = call-poly "get control reference by name.vi"("error in (no error)"=w545, "Control name"="guardar_Vref" ("String"), "Control references"=w530) -> ("error out"=w532:errorcluster, "Ctl Refnum"=w550:refnum<vi>)  [unwired: 3 in]
        n232 = Build Array(w550) -> (w549:refnum<vi>[])
        n233 = call "_get mutiple control reference by name.vi"("error in (no error)"=w532, "Control names"=string[] ["genera3", "knobFrec"] ("tipo_ciclo"), "Control references"=w530) -> ("error out"=w531:errorcluster, "References"=w533:refnum<vi>[])  [unwired: 3 in]
        n234 = call "Enable_Visible Buttons.vi"("Enable? (T)"=FALSE, "Controls Ref Array"=w549) -> ()  [unwired: 10 in]
        n235 = call "Enable_Visible Buttons.vi"("Enable? (T)"=TRUE, "Controls Ref Array"=w533) -> ()  [unwired: 10 in]
        n236 = disable-structure shown="Enabled" {
          disable-tunnel: [w555 w558] -> w536
          disable-tunnel: w531 -> [w554 w558]
          frame Disabled {
            n237 = property on="genera3" class="Bool (strict)"(error in=w554, "DisabledEnum"=T4."Enabled" ("Disabled"), "Value"=FALSE ("genera3")) -> (error out=w555:errorcluster)  [unwired: 1 in, 1 out]
          }
          frame Enabled {
          }
        }
        n238 = local write "frecMon1"(w553) -> ()
        n239 = local write "voltMon1"(w553) -> ()
        n240 = local write "frecMon2"(w553) -> ()
        n241 = local write "voltMon2"(w553) -> ()
      }
      frame "guardaVref" {
        n242 = local read "AjusteAmp"() -> (w561:T1)
        n243 = Divide(x=w561, y=T1 1000.0) -> (x/y=→"Vref":T1)
        n244 = Number To Fractional String(number=w561, precision (6)=i16 1) -> (F-format string=w564:string)  [unwired: 2 in]
        n245 = Format Into String(format string="Se guardó Vref = %s mV", w564) -> (resulting string=w567:string)  [unwired: 2 in, 1 out]
        n246 = One Button Dialog(message=w567) -> ()  [unwired: 1 in, 1 out]
      }
      frame "guardaVref2" {
        n247 = local read "AjusteAmp2"() -> (w570:T1)
        n248 = Divide(x=w570, y=T1 1000.0) -> (x/y=→"Vref2":T1)
        n249 = Number To Fractional String(number=w570, precision (6)=i16 1) -> (F-format string=w573:string)  [unwired: 2 in]
        n250 = Format Into String(format string="Se guardó Vref = %s mV", w573) -> (resulting string=w576:string)  [unwired: 2 in, 1 out]
        n251 = One Button Dialog(message=w576) -> ()  [unwired: 1 in, 1 out]
      }
      frame "Error" {
        w584 = T8 1 items=["no dialog", "OK message", "continue or stop message", "OK message + warnings", "continue/stop + warnings"] ("type of dialog (OK msg:1)")
        n252 = Variant To Data(error in=w580, type=errorcluster {"status"=FALSE, "code"=0, "source"=""} ("error out"), Variant=w577) -> (data=w582:errorcluster, error out=w581:errorcluster)
        n253 = call <vilib>:"Simple Error Handler.vi"("type of dialog (OK msg:1)"=w584, "error in (no error)"=w582) -> ()  [unwired: 3 in, 5 out]
        n254 = call-poly "Enqueue Message.vi"("error in (no error)"=w581, "Message"="Exit", "Message Queue"=w579) -> ("error out"=w578:errorcluster)  [unwired: 7 in, 1 out]
      }
      frame "----------------------Controles----------------------" {
      }
      frame "Exit" {
        w589 = TRUE
        # "#evangelio Manda a cerrar el EHL"
        # "#evangelio Manda a cerrar todos los Loops"
        n255 = Release Queue(queue=w595, error in (no error)=w596) -> (error out=w600:errorcluster)  [unwired: 1 in, 2 out]
        n256 = Unbundle By Name(w591) -> ("Control references"=w601:T7)
        n257 = for {
          tunnel: w594 -> [w604] mode=indexing
          tunnel: w592 -> [w603]
          tunnel: TRUE -> [w602]
          n258 = call-poly "Enqueue Message.vi"("Priority Message? (F)"=w602, "Message"=w603, "Message Queue"=w604) -> ()  [unwired: 7 in, 2 out]
        }
        n259 = call "Close All Ref.vi"("error in (no error)"=w600, "Control references"=w601) -> ("error out"=w598:errorcluster)  [unwired: 9 in]
        n260 = call "Fire User Event - Stop.vi"("error in (no error)"=w598, "Event Data"=w589, "User Event"="Exit EHL", "User Event in"=w593) -> ("error out"=w590:errorcluster)  [unwired: 7 in]
      }
      frame "Confirmar Salida" {
        n261 = Two Button Dialog(message="¿Quieres cerrar la aplicación?", 1:"No" ("T button name (\"OK\")"), 2:"Si" ("T button name (\"OK\")")) -> (T button?=w608:bool)
        n262 = case shown="True" w608 {
          tunnel: w607 -> [w613 w617]
          tunnel: [w613 w620] -> w605
          tunnel: w606 -> [_ w618]
          frame False {
          }
          frame True {
            n263 = call-poly "Enqueue Message.vi"("error in (no error)"=w617, "Message"="Detener_Instrumento", "Message Queue"=w618) -> ("error out"=w616:errorcluster, "dup Message Queue"=w615:refnum<queue>)  [unwired: 7 in]
            n264 = call-poly "Enqueue Message.vi"("error in (no error)"=w616, "Message"="Exit", "Message Queue"=w615) -> ("error out"=w620:errorcluster)  [unwired: 7 in, 1 out]
          }
        }
      }
      frame Default {
        n265 = xnode "Error Ring"("parameter 0"=w622) -> ("error out"=w621:errorcluster)
      }
    }
    n266 = call "Error Handler - Message Handling Loop.vi"("error in (no error)"=w125, "Message Queue"=w123) -> ("dup error in"=w124:errorcluster)  [unwired: 8 in, 1 out]
  }
  n267 = call "Inst_CNT90.vi"("error in"=w7, "All Message Queues in"=w8, "Prueba31 in"=w9) -> ()  [unwired: 8 in, 1 out]
  n268 = call "Inst_DS360.vi"("error in"=w7, "All Message Queues in"=w8, "Prueba09 in"=w9) -> ()  [unwired: 8 in, 1 out]
  n269 = call "Inst_K2002.vi"("error in"=w7, "All Message Queues in"=w8, "Prueba31 in"=w9) -> ()  [unwired: 8 in, 1 out]
  n270 = call-dynamic "CleanUp.vi"("Prueba09 in"=w4) -> ("error out"=w1:errorcluster, "Prueba09 out"=→"Prueba09 out":refnum<class "Prueba09.lvclass">)  [unwired: 9 in]
  n271 = Merge Errors(w22, w1, w2) -> (→"error out":errorcluster)
